vi "fromFileREAL.vi"(9 "increment":bool, 10 "Numeric":i32, 11 "MagAnalysis_Online in":refnum<class "MagAnalysis_Online.lvclass">) -> (1 "B [T]":dbl, 2 "Cluster":T1, 3 "MagAnalysis_Online out":refnum<class "MagAnalysis_Online.lvclass">, 4 "time":u32)   [LabVIEW 2020, in "MagAnalysis_Online.lvclass"]
uses:
  MagAnalysis_Online.lvclass
  fileCluster_TypDef.ctl
panel:
  in  "spec cluster 2":cluster{dbl[], dbl[]}[](array[cluster])
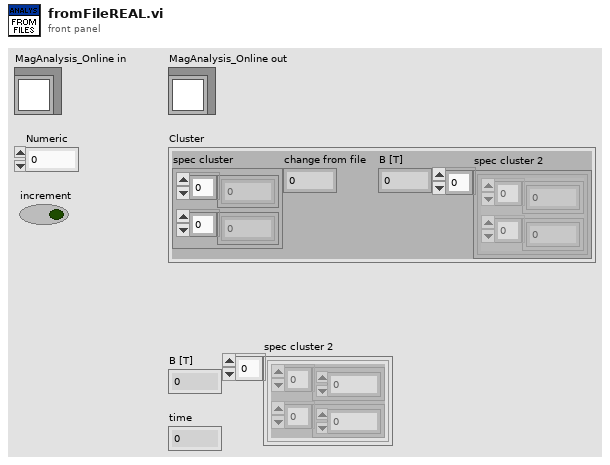
[diagram p1: front panel]
types:
  T1 = typedef "fileCluster_TypDef.ctl" = cluster{"spec cluster":cluster{dbl[], dbl[]}, "change from file":dbl, "B [T]":dbl, "spec cluster 2":cluster{dbl[], dbl[]}[]}
  T2 = typedef "MagAnalysis_Online.lvclass/analysis_data_typdef.ctl" = cluster{"cam0":T3, "cam1":T3, "cam2":T3, "cam3":T3}
  T3 = typedef "IMAQ Image.ctl" = refnum<image>
  T4 = typedef "bgImages_tyudef.ctl" = cluster{"cam 0":T3, "cam 1":T3, "cam 2":T3, "cam 3":T3}
  T5 = cluster{"spec cluster":cluster{dbl[], dbl[]}, "change from file":dbl, "B [T]":dbl, "spec cluster 2":cluster{dbl[], dbl[]}[]}
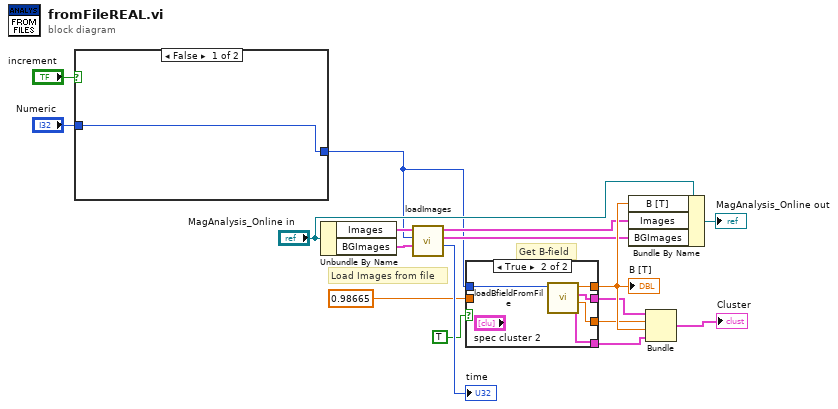
[diagram p0: block diagram]
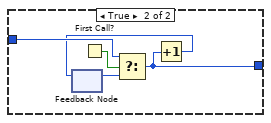
[diagram p2: hidden frame]
diagram:
  # "Get B-field"
  # "Load Images from file"
  n1 = case shown="False" "increment" {
    tunnel: "Numeric" -> [w18 w22]
    tunnel: [w18 w19] -> w2
    frame False {
    }
    frame True {
      n2 = feedback #1() -> (w20:i32)  [unwired: 1 in]
      n3 = First Call?() -> (First Call?: T/F=w23:bool)
      n4 = Select(t=w22, s=w23, f=w20) -> (s? t:f=w19:i32)
      n5 = Increment(x=w19) -> (x+1=w21:i32)
      n6 = feedback-in #1(w21) -> ()
    }
  }
  n7 = Unbundle By Name("MagAnalysis_Online in") -> ("Images"=w9:T2, "BGImages"=w10:T4)
  n8 = call "loadImages.vi"("BGImages"=w10, "Numeric"=w2, "data"=w9) -> ("time"=→"time":u32, "BG Images out"=w4:T4, "dat6a out"=w3:T2)  [unwired: 6 in]
  n9 = case shown="True" TRUE {
    tunnel: [w24 w29] -> w16
    tunnel: 0.98665 ("B [T] 2") -> [w24 _]
    tunnel: [_ w28] -> w14
    tunnel: [_ w27] -> w15
    tunnel: w2 -> [_ w26]
    tunnel: [_ w25] -> w1
    frame False {
    }
    frame True {
      n10 = call "loadBfieldFromFile.vi"("index"=w26) -> ("spec cluster 2"=w25:cluster{dbl[], dbl[]}[], "change from file"=w27:dbl, "spec cluster"=w28:cluster{dbl[], dbl[]}, "B [T]"=w29:dbl)  [unwired: 7 in]
    }
  }
  "B [T]" <- w16
  n11 = Bundle By Name(cluster="MagAnalysis_Online in", "B [T]"=w16, "Images"=w3, "BGImages"=w4) -> (→"MagAnalysis_Online out":refnum<class "MagAnalysis_Online.lvclass">)
  n12 = Bundle("spec cluster"=w14, "change from file"=w15, "B [T]"=w16, "spec cluster 2"=w1) -> (→"Cluster":T5)  [unwired: 1 in]
